vi "OpenWorkspaceManager.vi"(6 "Gateway IP Address (\"\": localhost)":string, 8 "error in (no error)":errorcluster, 11 "VeriStandTestCase in":refnum<class "VeriStandTestCase.lvclass">) -> (0 "error out":errorcluster, 3 "VeriStandTestCase out":refnum<class "VeriStandTestCase.lvclass">)   [LabVIEW 2016, in "VeriStandTestCase.lvclass"]
uses:
  VeriStandTestCase.lvclass
  VeriStandTestCase.lvclass/VeriStandTestCase.ctl
  VeriStandTestUtilities/VeriStandTestUtilities.lvlib
  <vilib>/NI VeriStand/Execution/Workspace/NI_VS Workspace ExecutionAPI.lvlib
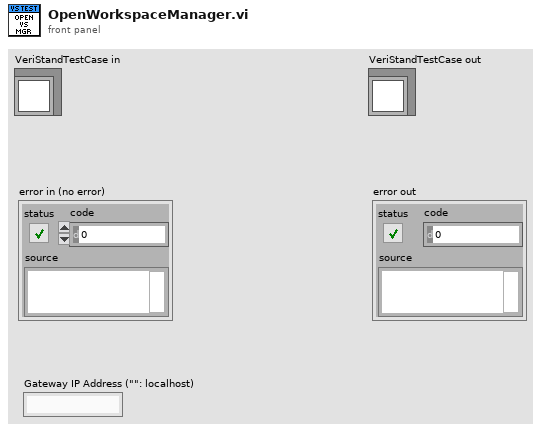
[diagram p1: front panel]
types:
  T1 = typedef "NI_VS Workspace ExecutionAPI.lvlib/WorkspaceAPI.ctl" = refnum<k24>
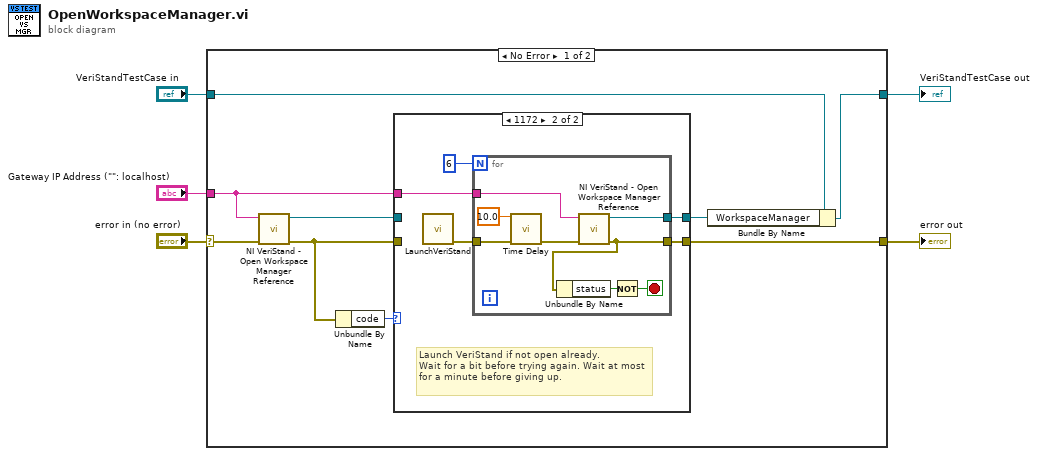
[diagram p0: block diagram]
diagram:
  n1 = case shown="No Error" "error in (no error)" {
    selector: "error in (no error)" -> [w6 w30]
    tunnel: [w14 w30] -> w5
    tunnel: [w13 w31] -> w4
    tunnel: "VeriStandTestCase in" -> [w10 w31]
    tunnel: "Gateway IP Address (\"\": localhost)" -> [w7 _]
    frame No Error {
      n2 = call <vilib>:"NI VeriStand - Open Workspace Manager Reference.vi"("error in (no error)"=w6, "Gateway IP Address (\"\": localhost)"=w7) -> ("error out"=w8:errorcluster, "WorkspaceManager"=w11:T1)  [unwired: 8 in]
      n3 = Unbundle By Name(w8) -> ("code"=w9:i32)
      n4 = case shown="1172" w9 {
        tunnel: w8 -> [w16 _]
        tunnel: [w16 w20] -> w14
        tunnel: w7 -> [_ w19]
        tunnel: w11 -> [w15 _]
        tunnel: [w15 w18] -> w12
        frame 0, Default {
        }
        frame 1172 {
          # "Launch VeriStand if not open already.\nWait for a bit before trying again. Wait at most for a minute before giving up."
          n5 = call "LaunchVeriStand.vi"() -> ("error out"=w21:errorcluster)  [unwired: 11 in]
          n6 = for {
            N: 6 -> [_]
            tunnel: w19 -> [w29]
            tunnel: [w28] -> w18
            tunnel: w21 -> [w26]
            tunnel: [w24] -> w20
            stop <- w22 stop-if-true
            n7 = call "Time Delay"("error in (no error)"=w26, "Delay Time (s)"=10.0) -> ("error out"=w25:errorcluster)  [unwired: 9 in]
            n8 = call <vilib>:"NI VeriStand - Open Workspace Manager Reference.vi"("error in (no error)"=w25, "Gateway IP Address (\"\": localhost)"=w29) -> ("error out"=w24:errorcluster, "WorkspaceManager"=w28:T1)  [unwired: 8 in]
            n9 = Unbundle By Name(w24) -> ("status"=w23:bool)
            n10 = Not(x=w23) -> (.not. x?=w22:bool)
          }
        }
      }
      n11 = Bundle By Name(cluster=w10, "WorkspaceManager"=w12) -> (w13:refnum<class "VeriStandTestCase.lvclass">)
    }
    frame Error {
    }
  }
  "error out" <- w5
  "VeriStandTestCase out" <- w4
